vi "SN R&W.vi"(7 "R/W":enum16{"R", "W"}(ring)=enum."W") -> (1 "添加的路径":path, 3 "SN":u32)   [LabVIEW 2011]
uses:
  C:/Program Files (x86)/National Instruments/LabVIEW 2011/resource/objmgr/daqmx.rc
panel:
  out "DevSerialNum":u32
  in  "path":path caption="路径"
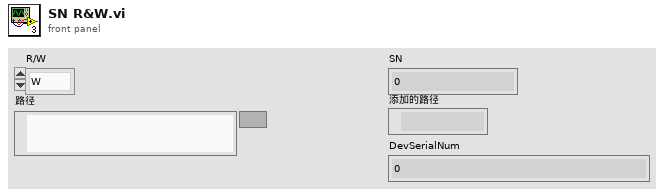
[diagram p1: front panel]
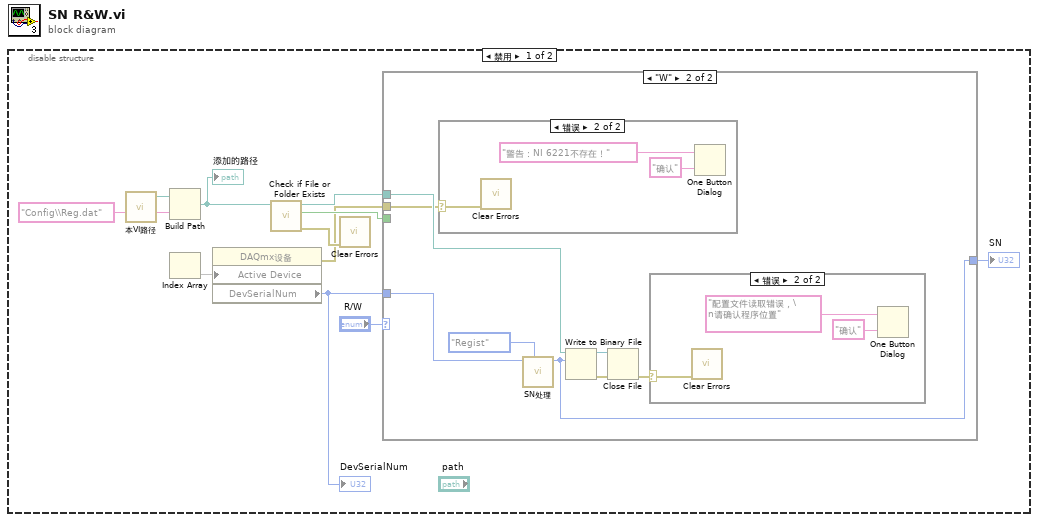
[diagram p0: block diagram]
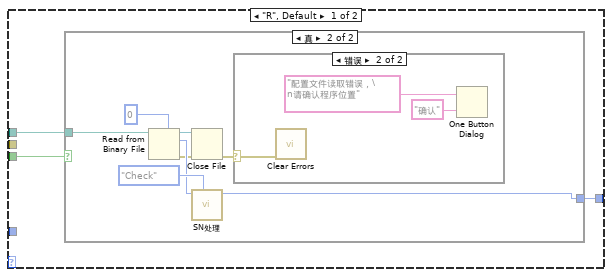
[diagram p2: hidden frame]
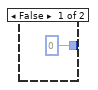
[diagram p3: hidden frame]
diagram:
  n1 = disable-structure shown="禁用" {
    frame Disabled {
      n2 = call "本VI路径.vi"() -> ("stripped path"=w1:path)  [unwired: 11 in]
      n3 = Build Path(base path=w1, name or relative path="Config\\Reg.dat" ("名称或相对路径")) -> (appended path=w2:path)
      "添加的路径" <- w2
      n4 = Index Array() -> (element=w6)  [unwired: 2 in]
      n5 = property class="DAQmx设备"("Active Device"=w6) -> (error out=w4:errorcluster, "DevSerialNum"=w5:u32)  [unwired: 2 in, 1 out]
      "DevSerialNum" <- w5
      n6 = call <vilib>:"Check if File or Folder Exists.vi"("path"=w2) -> ("error out"=w7:errorcluster, "file or folder exists?"=w9:bool, "dup path"=w10:path)  [unwired: 8 in]
      n7 = call <vilib>:"Clear Errors.vi"("error in (no error)"=w7) -> ()  [unwired: 6 in, 1 out]
      n8 = case shown="\"W\"" "R/W" {
        tunnel: [w14 w33] -> w8
        tunnel: w10 -> [w12 w34]
        tunnel: w9 -> [w13 _]
        tunnel: w5 -> [_ w28]
        tunnel: w4 -> [_ w27]
        frame "R", Default {
          n9 = case shown="真" w13 {
            tunnel: w12 -> [_ w22]
            tunnel: [u32 0 ("SN") w17] -> w14
            frame False {
            }
            frame True {
              n10 = Read from Binary File(5:0, 11:w22) -> (0:w18:errorcluster, 2:w20:i32, 3:w19:refnum<file>)  [unwired: 4 in, 1 out]
              n11 = Close File(refnum=w19, error in=w18) -> (error out=w16:errorcluster)  [unwired: 1 out]
              n12 = call "SN处理.vi"("动作"=enum16{"Check", "Regist"}."Check", "SN号"=w20) -> ("SN"=w17:u32)  [unwired: 9 in]
              n13 = case shown="错误" w16 {
                selector: w16 -> [_ w25]
                frame No Error {
                }
                frame Error {
                  n14 = call <vilib>:"Clear Errors.vi"("error in (no error)"=w25) -> ()  [unwired: 6 in, 1 out]
                  n15 = One Button Dialog(message="配置文件读取错误，\n请确认程序位置" ("消息"), button name ("OK")="确认" ("按钮名称（“确定”）")) -> ()  [unwired: 1 out]
                }
              }
            }
          }
        }
        frame "W" {
          n16 = case shown="错误" w27 {
            selector: w27 -> [_ w37]
            frame No Error {
            }
            frame Error {
              n17 = call <vilib>:"Clear Errors.vi"("error in (no error)"=w37) -> ()  [unwired: 6 in, 1 out]
              n18 = One Button Dialog(message="警告：NI 6221不存在！" ("消息"), button name ("OK")="确认" ("按钮名称（“确定”）")) -> ()  [unwired: 1 out]
            }
          }
          n19 = call "SN处理.vi"("动作"=enum16{"Check", "Regist"}."Regist", "SN号"=w28) -> ("SN"=w33:u32)  [unwired: 9 in]
          n20 = Write to Binary File(file (use dialog)=w34, data=w33) -> (refnum out=w31:refnum<file>, error out=w30:errorcluster)  [unwired: 4 in, 1 out]
          n21 = Close File(refnum=w31, error in=w30) -> (error out=w29:errorcluster)  [unwired: 1 out]
          n22 = case shown="错误" w29 {
            selector: w29 -> [_ w39]
            frame No Error {
            }
            frame Error {
              n23 = call <vilib>:"Clear Errors.vi"("error in (no error)"=w39) -> ()  [unwired: 6 in, 1 out]
              n24 = One Button Dialog(message="配置文件读取错误，\n请确认程序位置" ("消息"), button name ("OK")="确认" ("按钮名称（“确定”）")) -> ()  [unwired: 1 out]
            }
          }
        }
      }
      "SN" <- w8
    }
    frame Enabled {
    }
  }
